vi "Autocycle v0.51.vi"(7 "Message Queue":refnum<queue>, 8 "error in":errorcluster, 10 "All Para":cluster{"Auto Para":T1, "General Para":T2}={"Auto Para"={"Agitator Delays"=[], "TF Delays"=[], "Insertion Delays"=[], "Cutting Delays"=[], "PF Delays"=[], "Measur. Delays"=[], "Reject Delays"=[1000], "BF Delays"=[1000]}, "General Para"={"Max. Cons."=5.0, "Offset 1"=0.0, "Offset 2"=0.0, "Offset 3"=0.0, "Offset 4"=0.0, "OutputPause"=0.0, "RejectPause"=0.0}}) -> (0 "error out":errorcluster)   [LabVIEW 2017]
doc: "v0.5:\n- Skip Cutting on frst iteration\n\nv0.3:\n- Added End Cycle & Stop initiated as different stops\n- Make PF & TF not run on the first iteration"
uses:
  support/Message Queue/Message Cluster.ctl
  Controls/Auto Delays.ctl
  support/Controls/General Para.ctl
  Controls/Auto Times.ctl
  Global Variables/RT GV.vi
  Global Variables/FPGA GV.vi
  <vilib>/Utility/error.llb/Error Cluster From Error Code.vi
  <vilib>/rvi/errors/niLvFpgaAdjustHostInterfaceError.vi
  support/Message Queue/Enqueue Message (Single).vi
  <vilib>/rvi/interface/nirviReadWriteControl/nirviReadWriteControl.xnode
  Controls/FPGA Ref.ctl
  NiFpgaLv.dll
  <vilib>/rvi/interface/Simulation/niFpgaSimulationCallBeginRW.vi
  support/Message Queue/Message Queue.lvlib
panel:
  in  "EnableSOL":bool=TRUE
  out "Iterations to ON":i32
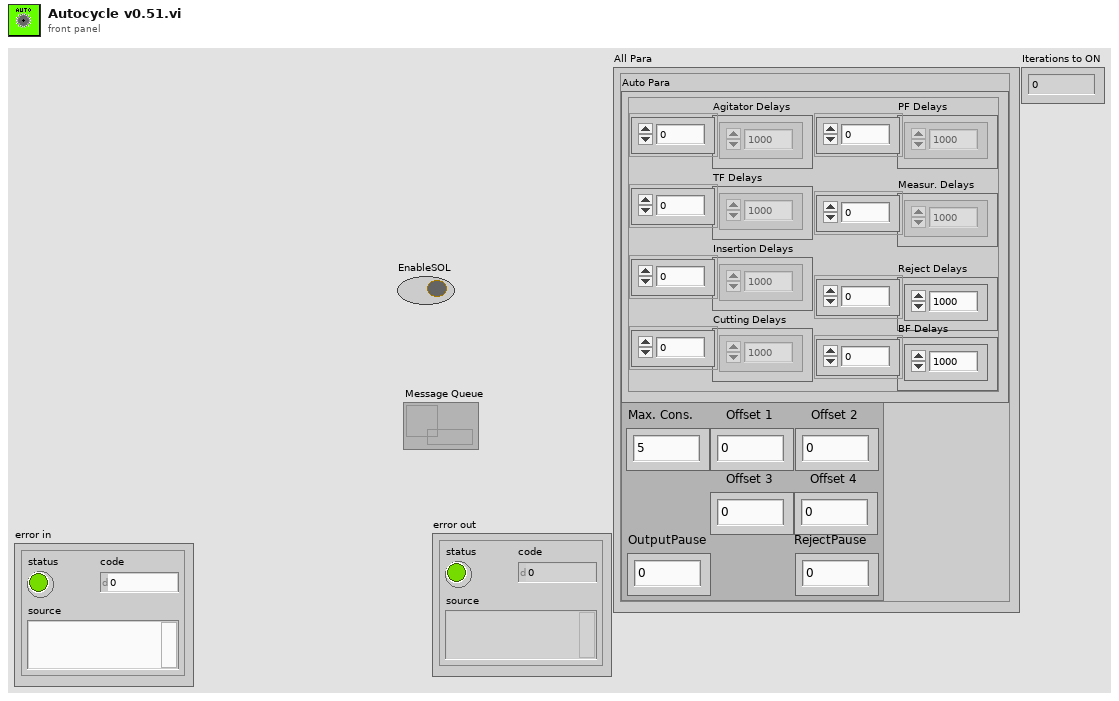
[diagram p1: front panel]
types:
  T1 = typedef "Auto Delays.ctl" = cluster{"Agitator Delays":u32[], "TF Delays":u32[], "Insertion Delays":u32[], "Cutting Delays":u32[], "PF Delays":u32[], "Measur. Delays":dbl[], "Reject Delays":u32[], "BF Delays":u32[]}
  T2 = typedef "General Para.ctl" = cluster{"Max. Cons.":dbl, "Offset 1":dbl, "Offset 2":dbl, "Offset 3":dbl, "Offset 4":dbl, "OutputPause":dbl, "RejectPause":dbl}
  T3 = typedef "FPGA Ref.ctl" = refnum<k20>
  T4 = cluster{"TL_Red":bool, "TL_Orange":bool, "TL_Green":bool, "TL_Buzzer":bool, "SOL_Index_Rotary_CW":bool, "SOL_Index_CNVR_Rotary_CCW":bool, "SOL_Index_CNVR_Stopper_Rear":bool, "SOL_Index_CNVR_Output _Separator _Rear":bool, "Bowl Feeder_ ON1":bool, "Pump_CNVR_Motor _ON":bool, "SOL_PC_Gating_CYL_Rear":bool, "SOL_Tube_Feed_Agitatator":bool, "SOL_Tube_Feed_Gating_CYL":bool, "SOL_Insertion _CYL":bool, "SOL_Insertion_Clamp_CYL":bool, "SOL_Cutting_CYL":bool, "SOL_Cutting_Clamp_CYL":bool, "SOL_Insertion_Air_Nozzle":bool, "SOL_Measurement_CYL":bool, "DO1.19":bool, "SOL_Rejection CYL_1":bool, "SOL_Rejection CYL_2":bool, "SOL_Rejection CYL_3":bool, "SOL_Rejection CYL_4":bool, "Bowl Feeder_ON2":bool, "SOL_BF_BlowerON":bool, "SOL_BF1_Track1":bool, "SOL_BF1_Track2":bool, "SOL_BF2_Track1":bool, "SOL_BF2_Track2":bool, "DO1.30":bool, "DO1.31":bool}
  T5 = typedef "Auto Times.ctl" = cluster{"Index Time":u32, "TF Time":u32, "Insertion Time":u32, "Cutting Time":u32, "PF Time":u32, "Meas. Time":u32, "Reject Time":u32}
  T6 = cluster{"Reject 1":bool, "Reject 2":bool, "Reject 3":bool, "Reject 4":bool}
  T7 = cluster{"Tube Present":bool[], "Parts Count":u32}
  T8 = cluster{"seconds since 1Jan1904":timestamp, "Auto Times":T5, "Tube Present":bool[], "Reject Pallets":cluster{"Reject 1":bool, "Reject 2":bool, "Reject 3":bool, "Reject 4":bool}, "Measurements":cluster{"1":dbl, "2":dbl, "3":dbl, "4":dbl}}
  T9 = typedef "Auto Stats.ctl" = cluster{"Time-Stamp":timestamp, "Auto Times":T5, "Measurements":cluster{"1":dbl, "2":dbl, "3":dbl, "4":dbl}, "Outputs":cluster{"Good Parts":u32, "Reject Parts":u32}, "Cycle Time":dbl, "Remarks":string}
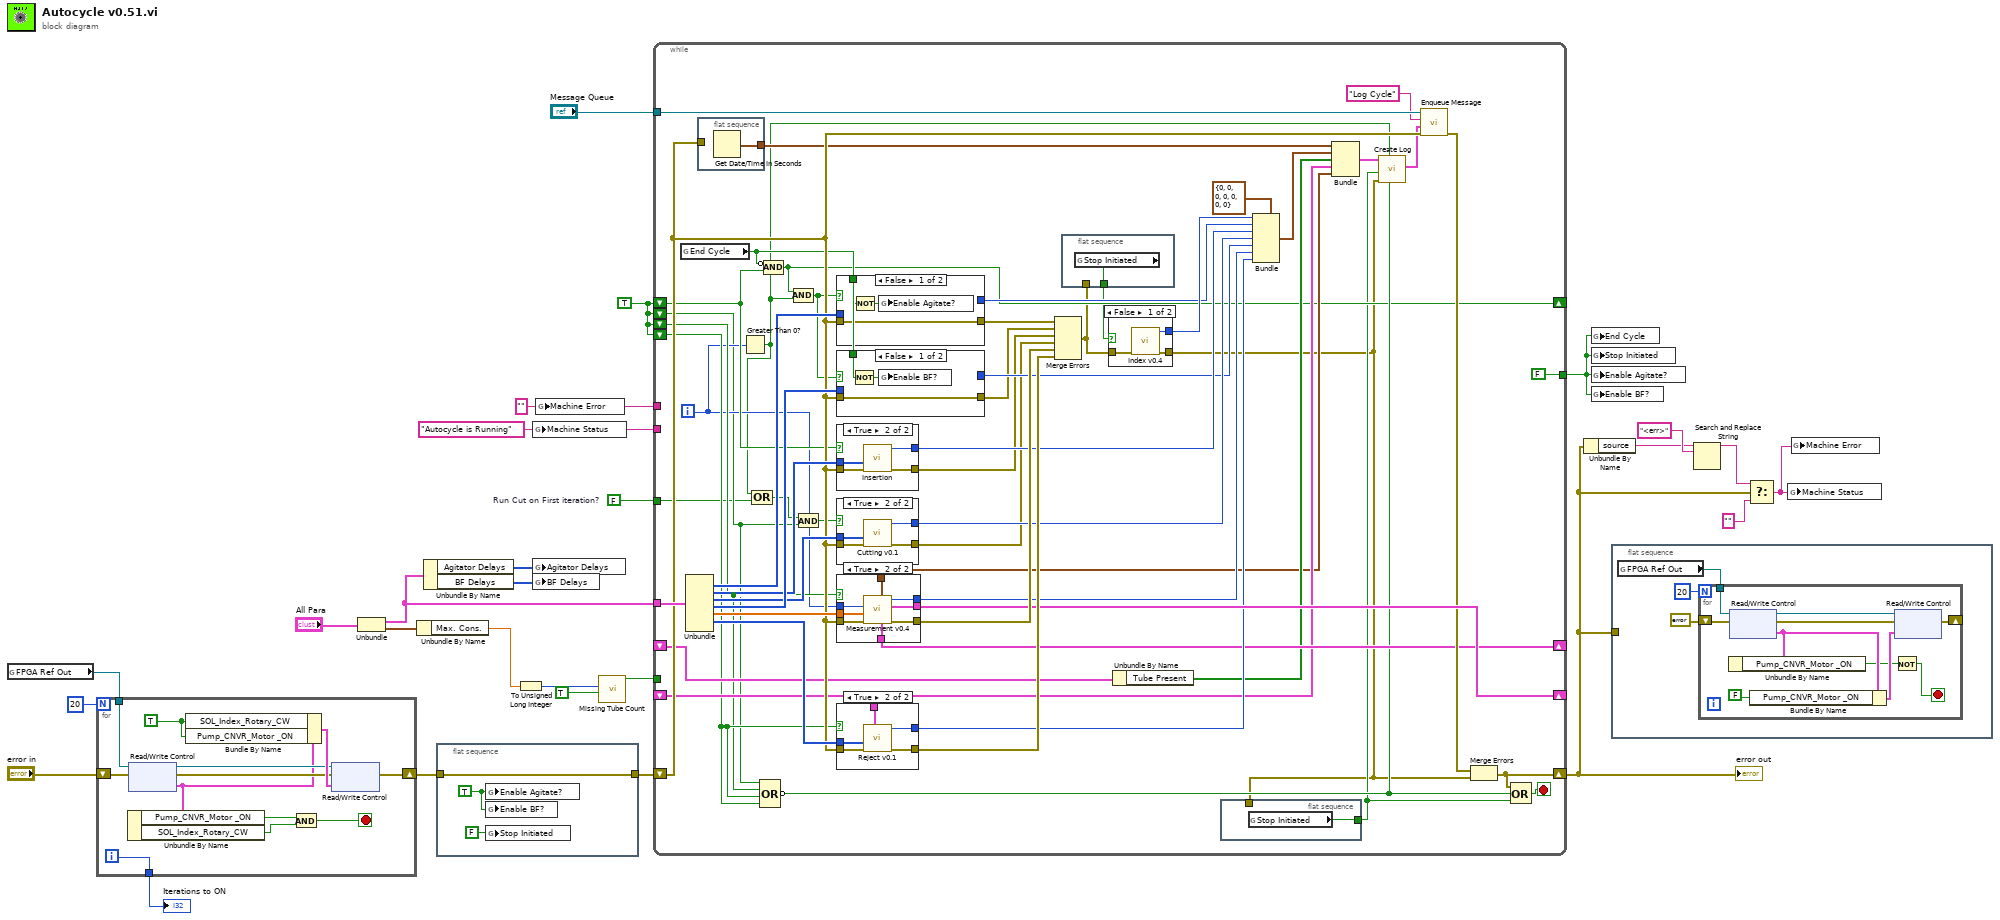
[diagram p0: block diagram]
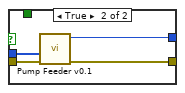
[diagram p3: hidden frame]
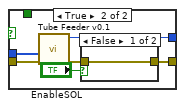
[diagram p6: hidden frame]
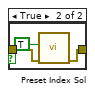
[diagram p7: hidden frame]
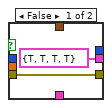
[diagram p9: hidden frame]
diagram:
  w1 = FALSE  # Run Cut on First iteration?
  w15 = "" ("Machine Error")
  w22 = "Autocycle is Running" ("Machine Status")
  w9 = TRUE
  n1 = global read "FPGA GV.vi" "FPGA Ref Out"() -> (w25:T3)
  n2 = for {
    N: 20 -> [_]
    tunnel: w25 -> [w39]
    shift-right: [w34] -> w12
    shift-left: "error in" -> [w35]
    tunnel: [w28] -> w2
    i -> [w28]
    stop <- w30 stop-if-true
    w31 = TRUE ("Pump_CNVR_Motor _ON")
    n3 = xnode "Read/Write Control"("FPGA VI Reference In"=w39, "error in"=w35) -> ("FPGA VI Reference Out"=w36:T3, "error out"=w37:errorcluster, "DO 1"=w33:T4)
    n4 = Unbundle By Name(w33) -> ("Pump_CNVR_Motor _ON"=w32:bool, "SOL_Index_Rotary_CW"=w29:bool)
    n5 = Bundle By Name(cluster=w33, "SOL_Index_Rotary_CW"=w31, "Pump_CNVR_Motor _ON"=w31) -> (w38:T4)
    n6 = Compound Arithmetic op=AND(w32, w29) -> (w30:bool)
    n7 = xnode "Read/Write Control"("FPGA VI Reference In"=w36, "error in"=w37, "DO 1"=w38) -> ("error out"=w34:errorcluster)  [unwired: 1 out]
  }
  "Iterations to ON" <- w2
  n8 = Unbundle("All Para") -> ("Auto Para"=w6:T1, "General Para"=w5:T2)
  n9 = Unbundle By Name(w5) -> ("Max. Cons."=w4:dbl)
  n10 = Unbundle By Name(w6) -> ("Agitator Delays"=w27:u32[], "BF Delays"=w26:u32[])
  n11 = flat-sequence {
    tunnel: [w42] -> w11
    tunnel: w12 -> [w42]
    frame #0 {
      w41 = TRUE ("Enable Agitate?")
      n12 = global write "RT GV.vi" "Enable Agitate?"(w41) -> ()
      n13 = global write "RT GV.vi" "Enable BF?"(w41) -> ()
      n14 = global write "RT GV.vi" "Stop Initiated"(FALSE ("Stop Initiated")) -> ()
    }
  }
  n15 = To Unsigned Long Integer(number=w4) -> (unsigned 32bit integer=w3:u32)
  n16 = global write "RT GV.vi" "Machine Status"(w22) -> ()
  n17 = global write "RT GV.vi" "Agitator Delays"(w27) -> ()
  n18 = global write "RT GV.vi" "BF Delays"(w26) -> ()
  n19 = global write "RT GV.vi" "Machine Error"(w15) -> ()
  n20 = call "Missing Tube Count.vi"("ResetMT?"=TRUE, "Max Successive"=w3) -> ("Boolean"=w13:bool)  [unwired: 8 in, 1 out]
  n21 = while {
    tunnel: w6 -> [w93]
    shift-right: [w70] -> w20
    shift-left: w11 -> [w71]
    shift-right: [w87] -> _
    shift-left: _ -> [w62]
    shift-right: [w54] -> _
    shift-left: w9 -> [w55]
    shift-left: w9 -> [w47]
    shift-left: w9 -> [w56]
    shift-left: w9 -> [w57]
    tunnel: "Message Queue" -> [w77]
    tunnel: [FALSE] -> w8
    tunnel: w22 -> [_]
    tunnel: w15 -> [_]
    shift-right: [w65] -> _
    shift-left: _ -> [w64]
    tunnel: w13 -> [_]
    tunnel: w1 -> [w44]
    i -> [w51]
    stop <- w86 stop-if-true
    n22 = global read "RT GV.vi" "End Cycle"() -> (w58:bool)
    n23 = Unbundle(w93) -> ("TF Delays"=w96:u32[], "Insertion Delays"=w95:u32[], "Cutting Delays"=w94:u32[], "PF Delays"=w97:u32[], "Measur. Delays"=w91:dbl[], "Reject Delays"=w89:u32[])  [unwired: 2 out]
    n24 = flat-sequence {
      tunnel: w71 -> [_]
      tunnel: [w104] -> w67
      frame #0 {
        n25 = Get Date/Time In Seconds() -> (seconds since 1Jan1904=w104:timestamp)
      }
    }
    n26 = Greater Than 0?(x=w51) -> (x > 0?=w43:bool)
    n27 = Compound Arithmetic op=OR(w43, w44) -> (w45:bool)
    n28 = Compound Arithmetic op=OR(w47, w56, w57, w57) -> (invert w60:bool)
    n29 = Compound Arithmetic op=AND(invert w58, w55) -> (w54:bool)
    n30 = Compound Arithmetic op=AND(w54, w43) -> (w53:bool)
    n31 = Compound Arithmetic op=AND(w45, w47) -> (w46:bool)
    n32 = case shown="False" w53 {
      tunnel: w71 -> [w124 w130]
      tunnel: [w124 w126] -> w92
      tunnel: w96 -> [_ w129]
      tunnel: [_ w128] -> w84
      tunnel: w58 -> [w123 _]
      frame False {
        n33 = Not(x=w123) -> (.not. x?=w122:bool)
        n34 = global write "RT GV.vi" "Enable Agitate?"(w122) -> ()
      }
      frame True {
        n35 = call "Tube Feeder v0.1.vi"("error in (no error)"=w130, "TF Para"=w129) -> ("error out"=w127:errorcluster, "TF Time"=w128:u32)  [unwired: 8 in]
        n36 = case shown="False" "EnableSOL" {
          tunnel: w127 -> [w131 w134]
          tunnel: [w131 w133] -> w126
          frame False {
          }
          frame True {
            n37 = call "Preset Index Sol.vi"("error in"=w134, "CCW?"=TRUE) -> ("error out"=w133:errorcluster)  [unwired: 9 in]
          }
        }
      }
    }
    n38 = case shown="False" w53 {
      tunnel: w71 -> [w107 w111]
      tunnel: [w107 w110] -> w73
      tunnel: w97 -> [_ w109]
      tunnel: [_ w108] -> w81
      tunnel: w58 -> [w106 _]
      frame False {
        n39 = Not(x=w106) -> (.not. x?=w105:bool)
        n40 = global write "RT GV.vi" "Enable BF?"(w105) -> ()
      }
      frame True {
        n41 = call "Pump Feeder v0.1.vi"("error in (no error)"=w111, "TF Delays"=w109) -> ("error out"=w110:errorcluster, "PF Time"=w108:u32)  [unwired: 8 in]
      }
    }
    n42 = case shown="True" w55 {
      tunnel: w71 -> [w117 w121]
      tunnel: [w117 w120] -> w74
      tunnel: w95 -> [_ w119]
      tunnel: [_ w118] -> w83
      frame False {
      }
      frame True {
        n43 = call "Insertion.vi"("error in (no error)"=w121, "Insertion Delays"=w119) -> ("error out"=w120:errorcluster, "Insertion Time"=w118:u32)  [unwired: 7 in, 1 out]
      }
    }
    n44 = case shown="True" w46 {
      tunnel: w71 -> [w112 w116]
      tunnel: [w112 w115] -> w75
      tunnel: w94 -> [_ w114]
      tunnel: [_ w113] -> w82
      frame False {
      }
      frame True {
        n45 = call "Cutting v0.1.vi"("error in (no error)"=w116, "Cutting Delays"=w114) -> ("error out"=w115:errorcluster, "Cutting Time"=w113:u32)  [unwired: 8 in]
      }
    }
    n46 = case shown="True" w56 {
      tunnel: w71 -> [w142 w150]
      tunnel: [w142 w149] -> w90
      tunnel: w91 -> [_ w148]
      tunnel: [_ w147] -> w80
      tunnel: [_ w146] -> w61
      tunnel: [T6 {"Reject 1"=TRUE, "Reject 2"=TRUE, "Reject 3"=TRUE, "Reject 4"=TRUE} ("Reject Pallets") w145] -> w87
      tunnel: [_ w144] -> w65
      tunnel: w51 -> [_ w143]
      frame False {
      }
      frame True {
        n47 = call "Measurement v0.4.vi"("error in (no error)"=w150, "TF Delays"=w148, "Loop Count"=w143) -> ("error out"=w149:errorcluster, "Reject Pallets"=w145:T6, "PF Time"=w147:u32, "Part Count"=w144:T7, "Measurements"=w146:cluster{"1":dbl, "2":dbl, "3":dbl, "4":dbl})  [unwired: 4 in]
      }
    }
    n48 = case shown="True" w57 {
      tunnel: w71 -> [w135 w140]
      tunnel: [w135 w139] -> w88
      tunnel: w89 -> [_ w138]
      tunnel: [_ w137] -> w79
      tunnel: w62 -> [_ w136]
      frame False {
      }
      frame True {
        n49 = call "Reject v0.1.vi"("Reject Pallets"=w136, "error in (no error)"=w140, "TF Delays"=w138) -> ("error out"=w139:errorcluster, "PF Time"=w137:u32)  [unwired: 7 in]
      }
    }
    n50 = Merge Errors(w92, w73, w74, w75, w90, w88) -> (w48:errorcluster)
    n51 = flat-sequence {
      tunnel: [w98] -> w49
      tunnel: w48 -> [_]
      frame #0 {
        n52 = global read "RT GV.vi" "Stop Initiated"() -> (w98:bool)
      }
    }
    n53 = case shown="False" w49 {
      tunnel: [w101 _] -> w85
      tunnel: w48 -> [w100 w102]
      tunnel: [w99 w102] -> w50
      frame False {
        n54 = call "Index v0.4.vi"("error in (no error)"=w100) -> ("error out"=w99:errorcluster, "Index Time"=w101:u32)  [unwired: 7 in, 2 out]
      }
      frame True {
      }
    }
    n55 = Unbundle By Name(w64) -> ("Tube Present"=w63:bool[])
    n56 = flat-sequence {
      tunnel: [w103] -> w52
      tunnel: w50 -> [_]
      frame #0 {
        n57 = global read "RT GV.vi" "Stop Initiated"() -> (w103:bool)
      }
    }
    n58 = Bundle(cluster=T5 {"Index Time"=0, "TF Time"=0, "Insertion Time"=0, "Cutting Time"=0, "PF Time"=0, "Meas. Time"=0, "Reject Time"=0} ("Auto Times"), "Index Time"=w85, "TF Time"=w84, "Insertion Time"=w83, "Cutting Time"=w82, "PF Time"=w81, "Meas. Time"=w80, "Reject Time"=w79) -> (w66:T5)
    n59 = Bundle("seconds since 1Jan1904"=w67, "Auto Times"=w66, "Tube Present"=w63, "Reject Pallets"=w62, "Measurements"=w61) -> (w59:T8)  [unwired: 1 in]
    n60 = call "Create Log.vi"("End Cycle?"=w60, "Not First Run?"=w43, "Error in"=w50, "Stop Initiated?"=w52, "Log Input Data"=w59) -> ("Auto Stats"=w68:T9)  [unwired: 6 in]
    n61 = call-poly "Enqueue Message.vi"("error in (no error)"=w71, "Message Data"=w68, "Message"="Log Cycle", "Message Queue"=w77) -> ("error out"=w69:errorcluster)  [unwired: 6 in, 1 out]
    n62 = Merge Errors(w69, w50) -> (w70:errorcluster)
    n63 = Compound Arithmetic op=OR(w70, w60, w52) -> (w86:bool)
  }
  "error out" <- w20
  n64 = Unbundle By Name(w20) -> ("source"=w18:string)
  n65 = global write "RT GV.vi" "End Cycle"(w8) -> ()
  n66 = global write "RT GV.vi" "Stop Initiated"(w8) -> ()
  n67 = global write "RT GV.vi" "Enable Agitate?"(w8) -> ()
  n68 = global write "RT GV.vi" "Enable BF?"(w8) -> ()
  n69 = flat-sequence {
    tunnel: w20 -> [_]
    frame #0 {
      n70 = global read "FPGA GV.vi" "FPGA Ref Out"() -> (w152:T3)
      n71 = for {
        N: 20 -> [_]
        tunnel: w152 -> [w163]
        shift-right: [w157] -> _
        shift-left: errorcluster {"status"=FALSE, "code"=0, "source"=""} ("error out") -> [w158]
        stop <- w154 stop-if-true
        n72 = xnode "Read/Write Control"("FPGA VI Reference In"=w163, "error in"=w158) -> ("FPGA VI Reference Out"=w159:T3, "error out"=w160:errorcluster, "DO 1"=w156:T4)
        n73 = Unbundle By Name(w156) -> ("Pump_CNVR_Motor _ON"=w155:bool)
        n74 = Bundle By Name(cluster=w156, "Pump_CNVR_Motor _ON"=FALSE) -> (w162:T4)
        n75 = Not(x=w155) -> (.not. x?=w154:bool)
        n76 = xnode "Read/Write Control"("FPGA VI Reference In"=w159, "error in"=w160, "DO 1"=w162) -> ("error out"=w157:errorcluster)  [unwired: 1 out]
      }
    }
  }
  n77 = Search and Replace String(input string=w18, search string="<err>") -> (result string=w17:string)  [unwired: 6 in, 3 out]
  n78 = Select(t=w17, s=w20, f="" ("Machine Status")) -> (s? t:f=w16:string)
  n79 = global write "RT GV.vi" "Machine Status"(w16) -> ()
  n80 = global write "RT GV.vi" "Machine Error"(w16) -> ()
